vi "16 and 8 pulses TX 8spc_ver2.vi"(7 "reset system clock":bool, 8 "referenses":T1={"clock x2"="IO Socket\\Data Clock 2x", "Memory In"="pulse on memory", "Memory In 2"="pulse on memory", "Memory In 3"="pulse on memory", "Memory In 4"="pulse on memory", "Memory In 5"="pulse on memory", "Memory In 6"="pulse on memory", "Memory In 7"="pulse on memory", "Memory In 8"="pulse on memory"}, 9 "IQ_run":bool=TRUE, 10 "PDW input Valid":bool, 11 "array PDW":u64[](array[numeric])=[0, 0, 0, 0]) -> (0 "trig out":bool, 1 "pulse TX status":T2, 2 "output valid":bool, 3 "IQ out":T3[](array[typedef]), 4 "ready for input":bool)   [LabVIEW 2021]
uses:
  <instrlib>/_niInstr/DSP/v1/Shared/Public/IQ Data.ctl
  pulse_tx_vis/CTL/mode_type.ctl
  <instrlib>/_niInstr/Basic Elements/v1/FPGA/Private/Count Up U64.vi
  <instrlib>/_niInstr/Basic Elements/v1/FPGA/Private/Count Up U32.vi
  <instrlib>/_niInstr/Basic Elements/v1/FPGA/niInstr Basic Elements v1 FPGA.lvlib
  <instrlib>/_niInstr/DSP/v1/Shared/niInstr DSP v1 Shared.lvlib
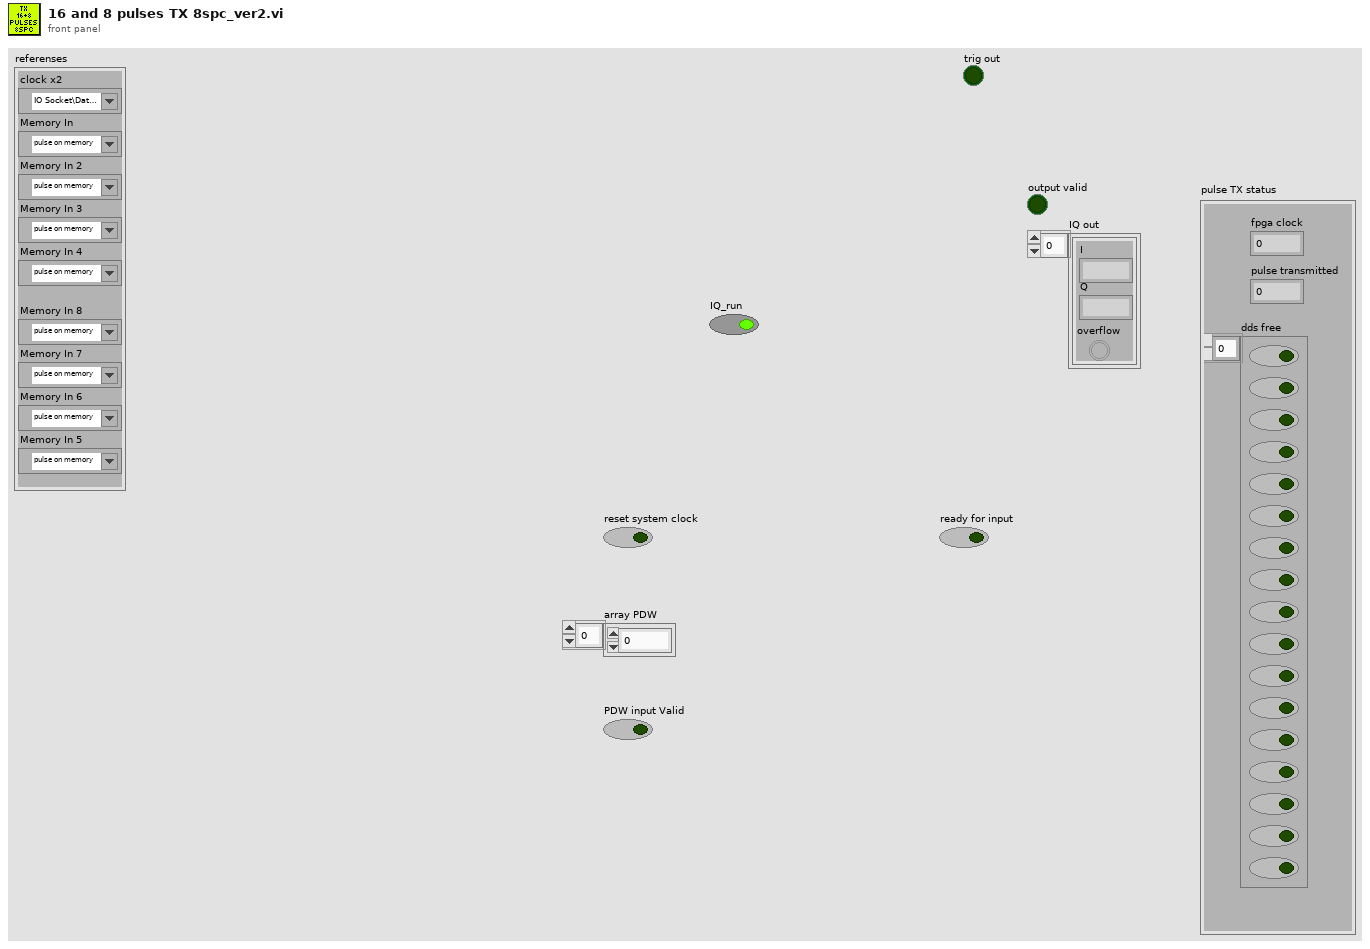
[diagram p1: front panel]
types:
  T1 = cluster{"clock x2":refnum<k21>, "Memory In":refnum<k21>, "Memory In 2":refnum<k21>, "Memory In 3":refnum<k21>, "Memory In 4":refnum<k21>, "Memory In 5":refnum<k21>, "Memory In 6":refnum<k21>, "Memory In 7":refnum<k21>, "Memory In 8":refnum<k21>}
  T2 = cluster{"fpga clock":u64, "pulse transmitted":u32, "dds free":bool[]}
  T3 = typedef "niInstr DSP v1 Shared.lvlib/IQ Data.ctl" = cluster{"I":fxp<+/-,18,1>, "Q":fxp<+/-,18,1>, "overflow":bool}
  T4 = cluster{"clock x2":refnum<k21>, "Memory In":refnum<k21>, "Memory In 2":refnum<k21>, "Memory In 3":refnum<k21>, "Memory In 4":refnum<k21>}
  T5 = typedef "mode_type.ctl" = enum8{"CW", "from memory 1", "NC - cw", "LFM", "BPSK", "QPSK"}
  T6 = typedef "pdw.ctl" = cluster{"PW":u32, "frequency shift":fxp<+/-,48,0>, "amp":fxp<+/-,18,1>, "mode type":T5, "mode depth":u32, "mode filter":u8, "phase shift":fxp<+/-,16,1>, "pulse shape filter":u8}
  T7 = cluster{"I":fxp<+/-,18,1>, "Q":fxp<+/-,18,1>, "overflow":bool}[]
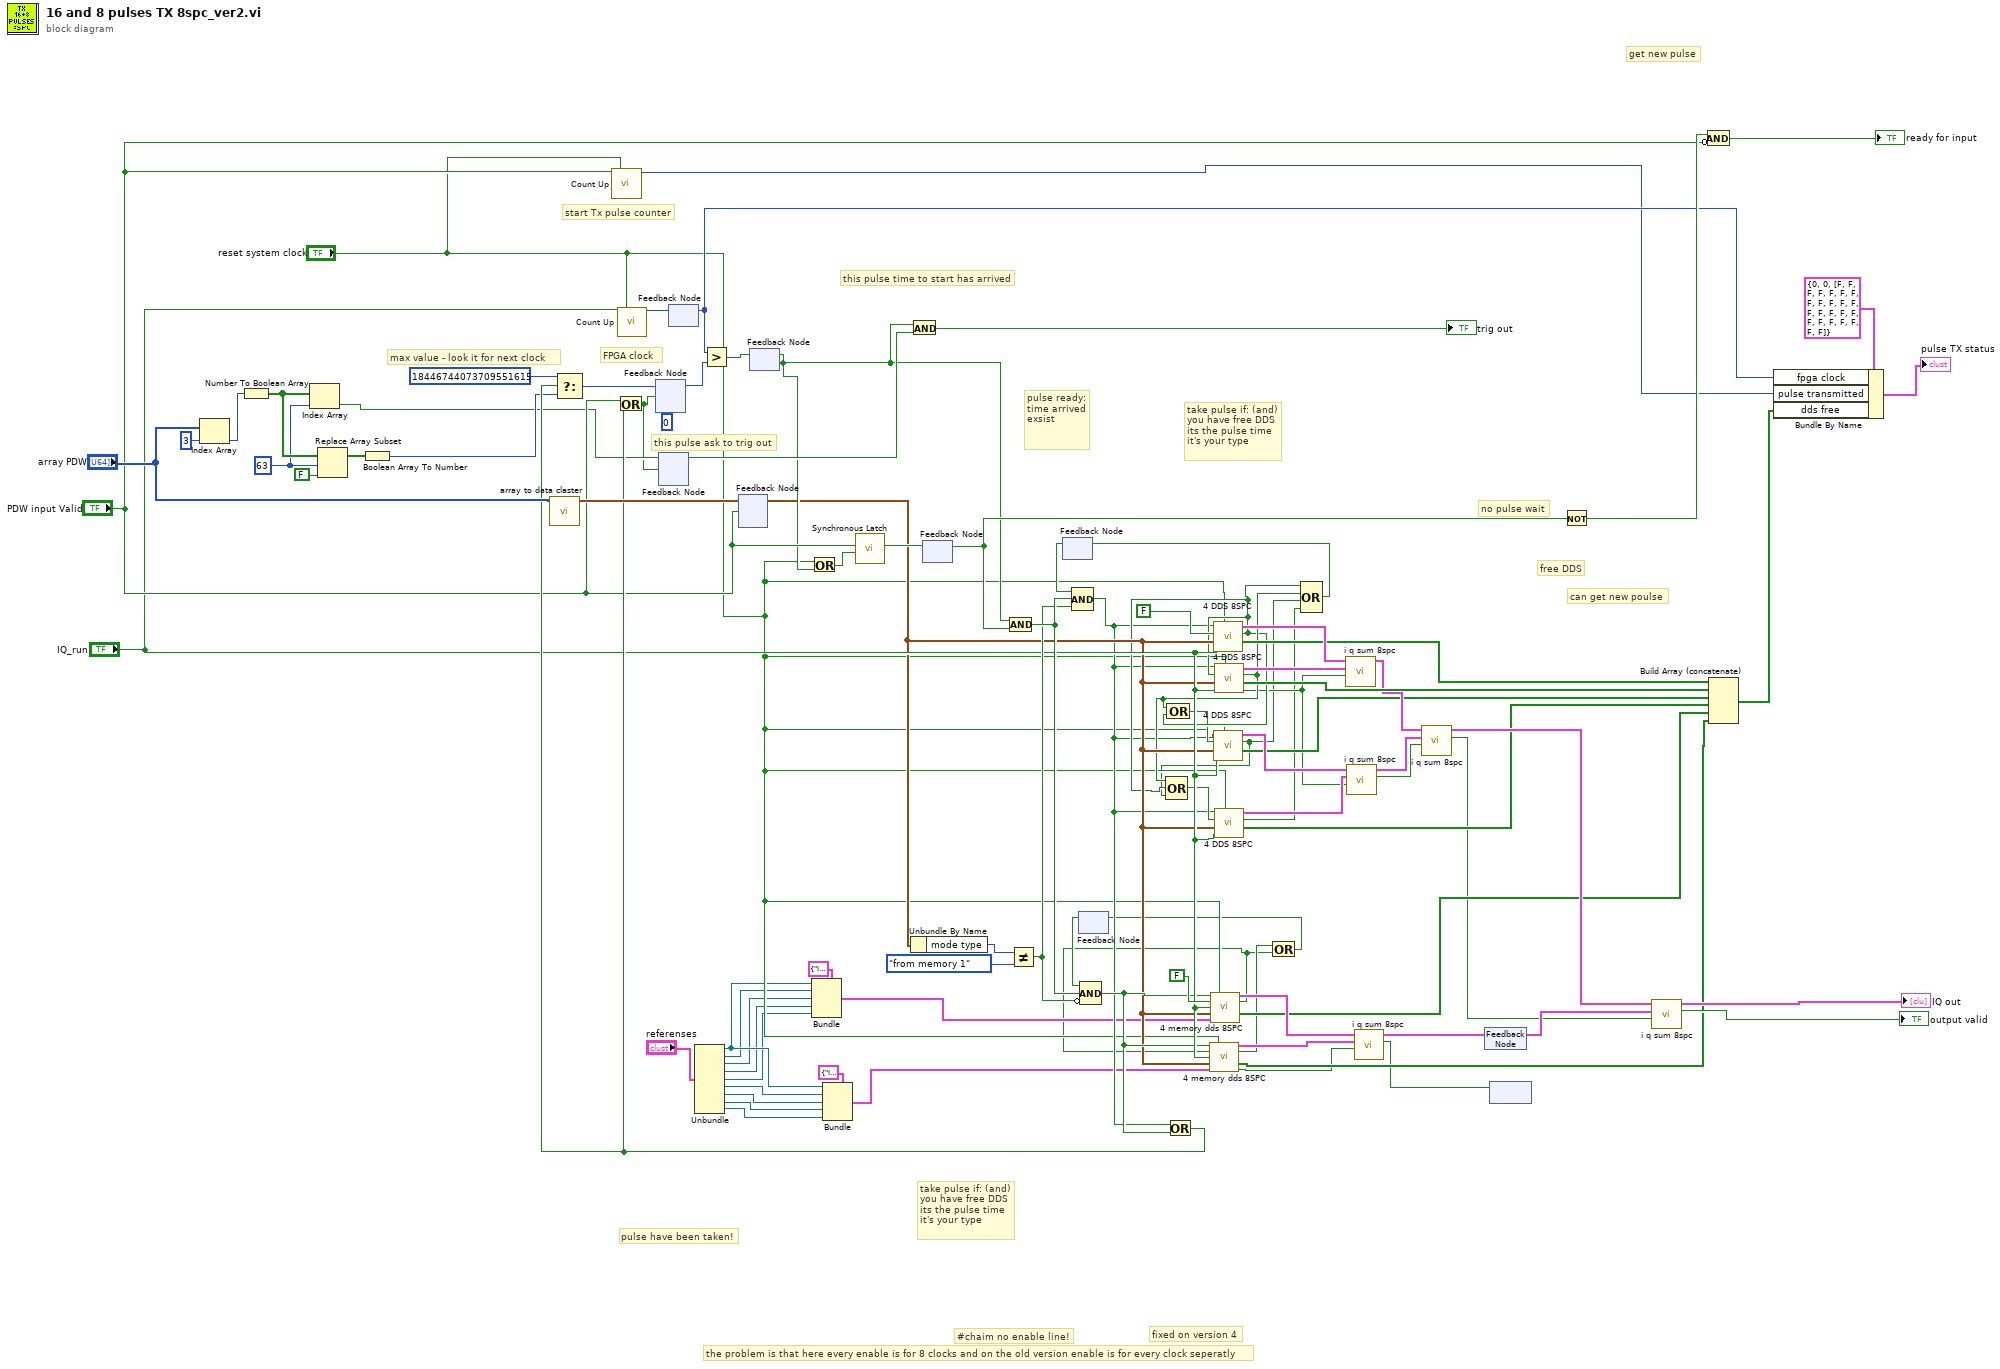
[diagram p0: block diagram]
diagram:
  w56 = 63 ("index")
  # "fixed on version 4"
  # "this pulse ask to trig out"
  # "pulse ready:\ntime arrived\nexsist"
  # "take pulse if: (and)\nyou have free DDS\nits the pulse time\nit's your type"
  # "take pulse if: (and)\nyou have free DDS\nits the pulse time\nit's your type"
  # "pulse have been taken!"
  # "the problem is that here every enable is for 8 clocks and on the old version enable is for every clock seperatly"
  # "#chaim no enable line!"
  # "start Tx pulse counter"
  # "FPGA clock"
  # "this pulse time to start has arrived"
  # "max value - look it for next clock"
  # "get new pulse"
  # "can get new poulse"
  # "no pulse wait"
  # "free DDS"
  n1 = Index Array(array="array PDW", index=3) -> (element=w58:u64)
  n2 = Number To Boolean Array(number=w58) -> (Boolean array=w57:bool[])
  n3 = Index Array(array=w57, index=w56) -> (element=w52:bool)
  n4 = Replace Array Subset(array=w57, new element=FALSE ("new element/subarray"), index=w56) -> (w54:bool[])
  n5 = Boolean Array To Number(Boolean array=w54) -> (number=w53:u64)
  n6 = call "array to data claster.vi"("Array"="array PDW") -> ("Cluster"=w75:T6)  [unwired: 10 in]
  n7 = call-poly <instrlib>:"Count Up.vi"("increment"="PDW input Valid", "reset"="reset system clock") -> ("count out"=w79:u32)  [unwired: 13 in]
  n8 = call-poly <instrlib>:"Count Up.vi"("increment"="IQ_run", "reset"="reset system clock") -> ("count out"=w89:u64)  [unwired: 13 in]
  n9 = feedback #1(u64 0 ("U64")) -> (w83:u64)
  n10 = feedback #2() -> (w50:bool)  [unwired: 1 in]
  n11 = feedback #3() -> (w80:u64)  [unwired: 1 in]
  n12 = feedback-in #3(w89) -> ()
  n13 = Unbundle("referenses") -> ("clock x2"=w24:refnum<k21>, "Memory In"=w23:refnum<k21>, "Memory In 2"=w22:refnum<k21>, "Memory In 3"=w21:refnum<k21>, "Memory In 4"=w20:refnum<k21>, "Memory In 5"=w19:refnum<k21>, "Memory In 6"=w18:refnum<k21>, "Memory In 7"=w17:refnum<k21>, "Memory In 8"=w16:refnum<k21>)
  n14 = Greater?(x=w80, y=w83) -> (0:w93:bool)
  n15 = feedback #4() -> (w36:T6)  [unwired: 1 in]
  n16 = feedback-in #4(w75, "PDW input Valid") -> ()
  n17 = feedback #5() -> (w49:bool)  [unwired: 1 in]
  n18 = feedback-in #5(w93) -> ()
  n19 = Or(x="reset system clock", y=w49) -> (x .or. y?=w62:bool)
  n20 = Bundle(cluster=T4 {"clock x2"="IO Socket\\Data Clock 2x", "Memory In"="pulse on memory", "Memory In 2"="pulse on memory", "Memory In 3"="pulse on memory", "Memory In 4"="pulse on memory"} ("referenses"), "clock x2"=w24, "Memory In"=w23, "Memory In 2"=w22, "Memory In 3"=w21, "Memory In 4"=w20) -> (w15:T4)
  n21 = Bundle(cluster=T4 {"clock x2"="IO Socket\\Data Clock 2x", "Memory In"="pulse on memory", "Memory In 2"="pulse on memory", "Memory In 3"="pulse on memory", "Memory In 4"="pulse on memory"} ("referenses"), "clock x2"=w24, "Memory In"=w19, "Memory In 2"=w18, "Memory In 3"=w17, "Memory In 4"=w16) -> (w14:T4)
  n22 = call <instrlib>:"Synchronous Latch.vi"("clear"=w62, "set"="PDW input Valid") -> ("out"=w60:bool)  [unwired: 9 in]
  n23 = And(x=w49, y=w50) -> (x .and. y?=→"trig out":bool)
  n24 = Unbundle By Name(w36) -> ("mode type"=w77:T5)
  n25 = feedback #6() -> (w59:bool)  [unwired: 1 in]
  n26 = feedback-in #6(w60) -> ()
  n27 = And(x=w49, y=w59) -> (x .and. y?=w72:bool)
  n28 = Not Equal?(x=w77, y=mode_type."from memory 1") -> (x != y?=w71:bool)
  n29 = feedback #7() -> (w68:bool)  [unwired: 1 in]
  n30 = Compound Arithmetic op=AND(w68, w72, w71) -> (w31:bool)
  n31 = feedback #8() -> (w5:bool)  [unwired: 1 in]
  n32 = Compound Arithmetic op=AND(w5, w72, invert w71) -> (w39:bool)
  n33 = Or(x=w31, y=w39) -> (x .or. y?=w69:bool)
  n34 = Select(t=u64 18446744073709551615, s=w69, f=w53) -> (s? t:f=w87:u64)
  n35 = Or(x="PDW input Valid", y=w69) -> (x .or. y?=w51:bool)
  n36 = feedback-in #1(w87, w51) -> ()
  n37 = feedback-in #2(w52, w51) -> ()
  n38 = call "4 memory dds 8SPC.vi"("new PDW in"=w39, "stop this pulse"="reset system clock", "free DDS before me?"=FALSE, "run"="IQ_run", "pdw in"=w36, "referenses"=w15) -> ("IQ out"=w42:T3[], "have free DDS"=w4:bool, "state of every DDS"=w38:bool[])  [unwired: 6 in, 1 out]
  n39 = call "4 memory dds 8SPC.vi"("new PDW in"=w39, "stop this pulse"="reset system clock", "free DDS before me?"=w4, "run"="IQ_run", "pdw in"=w36, "referenses"=w14) -> ("IQ out"=w41:T3[], "have free DDS"=w7:bool, "state of every DDS"=w37:bool[], "output valid"=w12:bool)  [unwired: 6 in]
  n40 = call "4 DDS 8SPC.vi"("clear DDS"="reset system clock", "input valid"="IQ_run", "pdw in"=w36, "free DDS before me?"=FALSE, "new PDW in"=w31) -> ("state of every DDS"=w64:bool[], "have free DDS"=w34:bool, "IQ out"=w67:T3[])  [unwired: 3 in, 1 out]
  n41 = call "4 DDS 8SPC.vi"("clear DDS"="reset system clock", "input valid"="IQ_run", "pdw in"=w36, "free DDS before me?"=w34, "new PDW in"=w31) -> ("output valid"=w13:bool, "state of every DDS"=w63:bool[], "have free DDS"=w35:bool, "IQ out"=w66:T3[])  [unwired: 3 in]
  n42 = Compound Arithmetic op=OR(w35, w34) -> (w32:bool)
  n43 = call "4 DDS 8SPC.vi"("clear DDS"="reset system clock", "input valid"="IQ_run", "pdw in"=w36, "free DDS before me?"=w32, "new PDW in"=w31) -> ("state of every DDS"=w28:bool[], "have free DDS"=w2:bool, "IQ out"=w47:T3[])  [unwired: 3 in, 1 out]
  n44 = Compound Arithmetic op=OR(w35, w34, w2) -> (w33:bool)
  n45 = call "4 DDS 8SPC.vi"("clear DDS"="reset system clock", "input valid"="IQ_run", "pdw in"=w36, "free DDS before me?"=w33, "new PDW in"=w31) -> ("state of every DDS"=w29:bool[], "have free DDS"=w1:bool, "IQ out"=w46:T3[])  [unwired: 3 in, 1 out]
  n46 = Compound Arithmetic op=OR(w7, w4) -> (w6:bool)
  n47 = feedback-in #8(w6) -> ()
  n48 = Compound Arithmetic op=OR(w34, w35, w2, w1) -> (w65:bool)
  n49 = feedback-in #7(w65) -> ()
  n50 = call "i q sum 8spc.vi"("input valid"=w13, "IQ in 2"=w66, "IQ in"=w67) -> ("IQ out"=w44:T7)  [unwired: 7 in, 1 out]
  n51 = call "i q sum 8spc.vi"("input valid"=w13, "IQ in 2"=w46, "IQ in"=w47) -> ("output valid"=w8:bool, "IQ out"=w45:T7)  [unwired: 7 in]
  n52 = call "i q sum 8spc.vi"("input valid"=w12, "IQ in 2"=w41, "IQ in"=w42) -> ("output valid"=w3:bool, "IQ out"=w11:T7)  [unwired: 7 in]
  n53 = call "i q sum 8spc.vi"("input valid"=w8, "IQ in 2"=w45, "IQ in"=w44) -> ("output valid"=w9:bool, "IQ out"=w43:T7)  [unwired: 7 in]
  n54 = feedback-in #9(w11) -> ()
  n55 = feedback #9() -> (w10:T7)  [unwired: 1 in]
  n56 = feedback #10() -> ()  [unwired: 2 in]
  n57 = feedback-in #10(w3) -> ()
  n58 = Not(x=w59) -> (.not. x?=w84:bool)
  n59 = call "i q sum 8spc.vi"("input valid"=w9, "IQ in 2"=w10, "IQ in"=w43) -> ("output valid"=→"output valid":bool, "IQ out"=→"IQ out":T7)  [unwired: 7 in]
  n60 = Compound Arithmetic op=AND(w84, invert "PDW input Valid") -> (→"ready for input":bool)
  n61 = Build Array (concatenate)(w64, w63, w28, w29, w38, w37) -> (w78:bool[])
  n62 = Bundle By Name(cluster=T2 {"fpga clock"=0, "pulse transmitted"=0, "dds free"=[FALSE, FALSE, FALSE, FALSE, FALSE, FALSE, FALSE, FALSE, FALSE, FALSE, FALSE, FALSE, FALSE, FALSE, FALSE, FALSE, FALSE, FALSE, FALSE, FALSE, FALSE, FALSE, FALSE, FALSE]} ("pulse TX status"), "fpga clock"=w80, "pulse transmitted"=w79, "dds free"=w78) -> (→"pulse TX status":T2)
